vi "Global Log To String.vi"(10 "Log":T1) -> (3 "Log String":string)   [LabVIEW 2017, in "Communicable State Machine.lvlib"]
doc: "Converts global log data clusters to strings.\n\n-- <b>Controls</b> --\n- <b>Log</b>: Global log data cluster.\n\n-- <b>Indicators</b> --\n- <b>Log String</b>: Global log string."
uses:
  Communicable State Machine.lvlib
  _Support/Typedef/_CSM_GlobalLog_MSG.ctl
  _Support/Typedef/_CSM_Response Source Message.ctl
  _Support/Typedef/_CSM_GlobalLog_MSG_TYPE.ctl
  _Shared/CSM Shared.lvlib
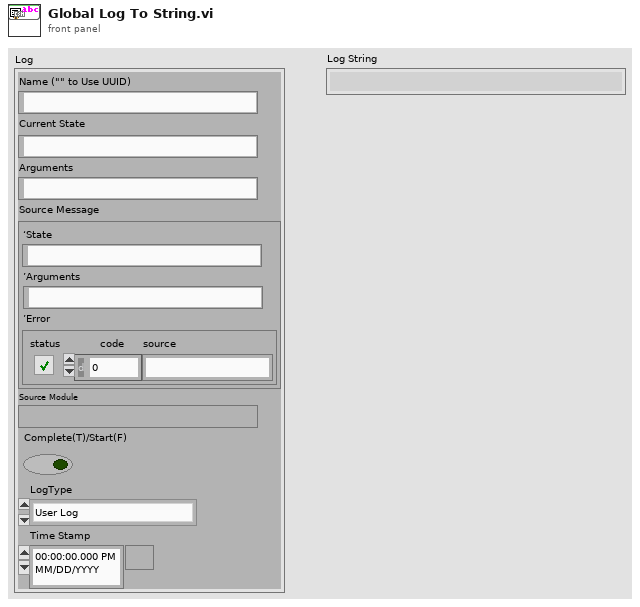
[diagram p1: front panel]
types:
  T1 = typedef "Communicable State Machine.lvlib/_CSM_GlobalLog_MSG.ctl" = cluster{"Name (\"\" to Use UUID)":string, "Current State":string, "Arguments":string, "Source Message":T2, "Source Module":string, "Complete(T)/Start(F)":bool, "LogType":T3, "Time Stamp":timestamp}
  T2 = typedef "Communicable State Machine.lvlib/_CSM_Response Source Message.ctl" = cluster{"‘State":string, "’Arguments":string, "’Error":errorcluster}
  T3 = typedef "Communicable State Machine.lvlib/_CSM_GlobalLog_MSG_TYPE.ctl" = enum16{"User Log", "State Change", "Status", "Interrupt", "Register", "Unregister", "Error Log", "Module Created", "Module Destroyed", "Async Message", "No-Rep Async Message", "Sync Message", "AsyncMsg Complete", "SyncMsg Complete"}
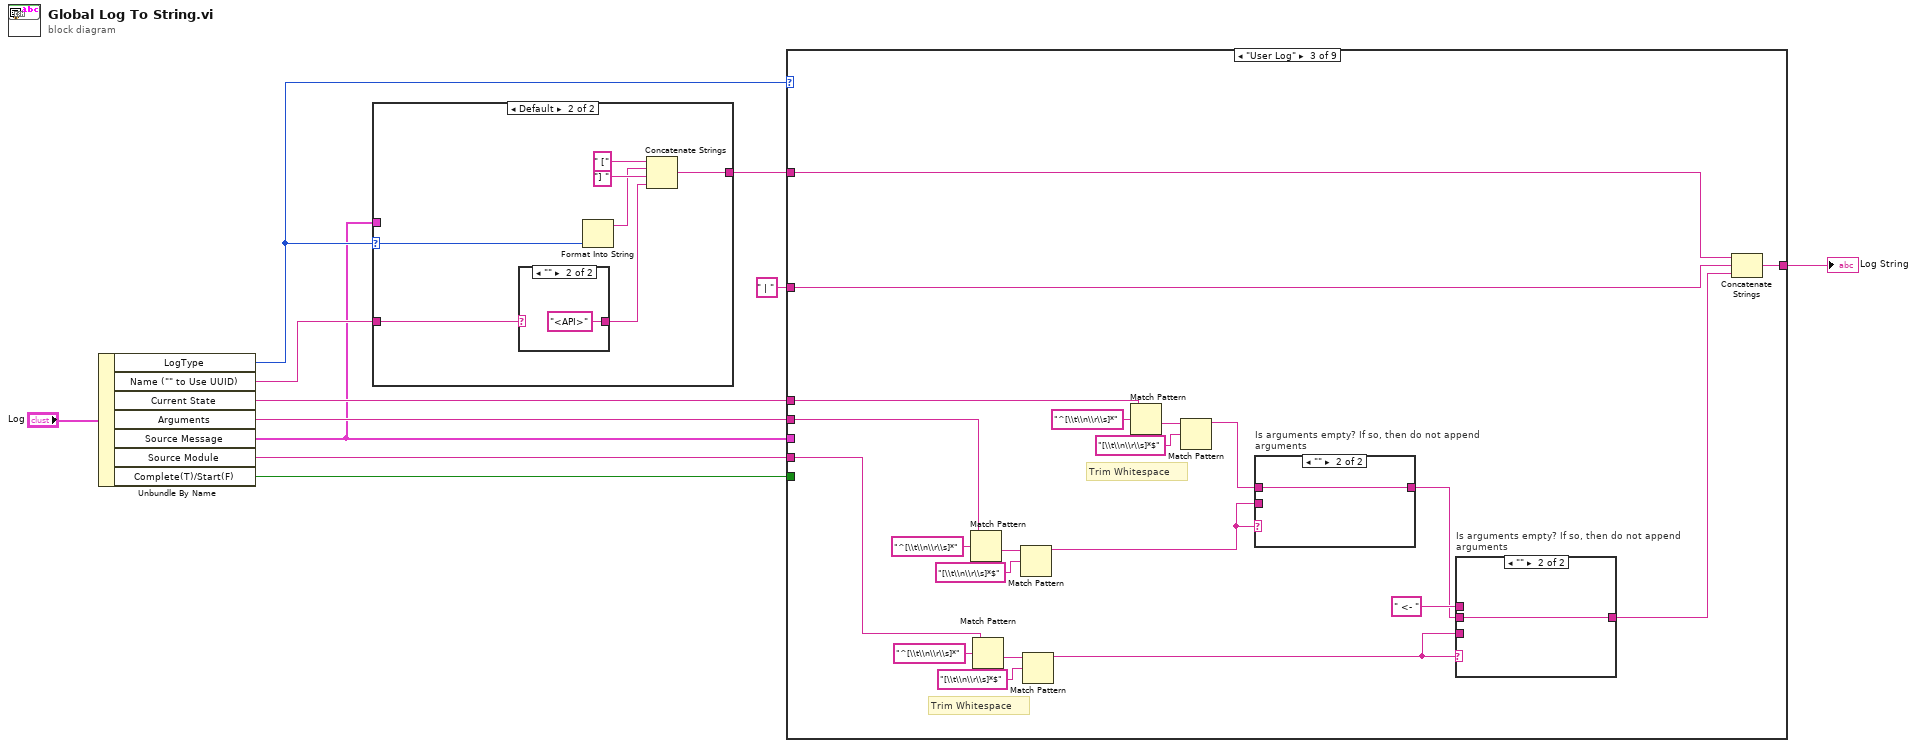
[diagram p0: block diagram]
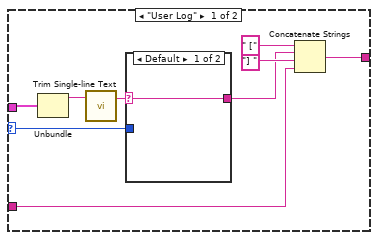
[diagram p2: hidden frame]
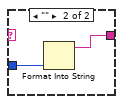
[diagram p3: hidden frame]
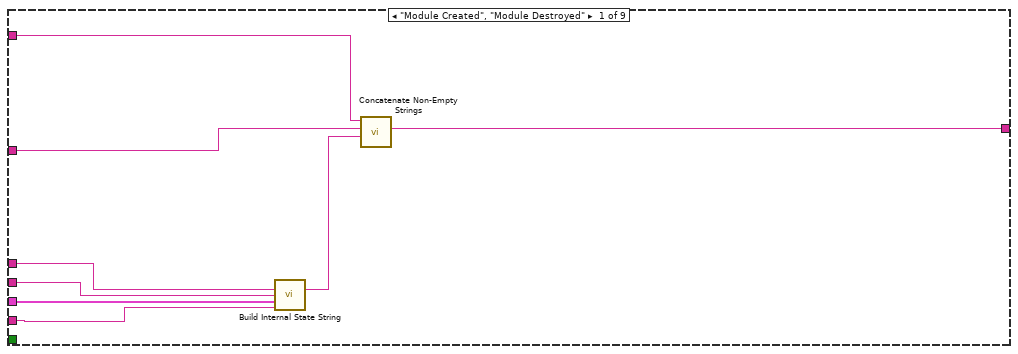
[diagram p5: hidden frame]
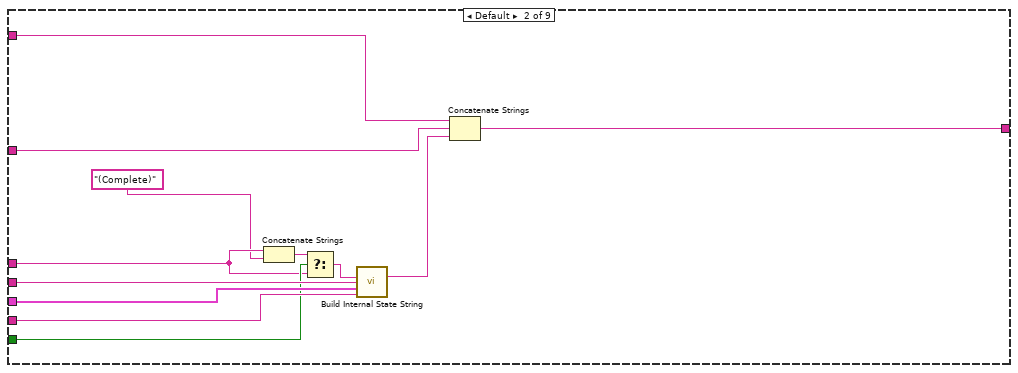
[diagram p6: hidden frame]
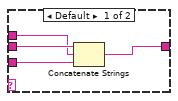
[diagram p7: hidden frame]
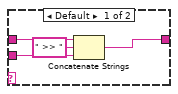
[diagram p8: hidden frame]
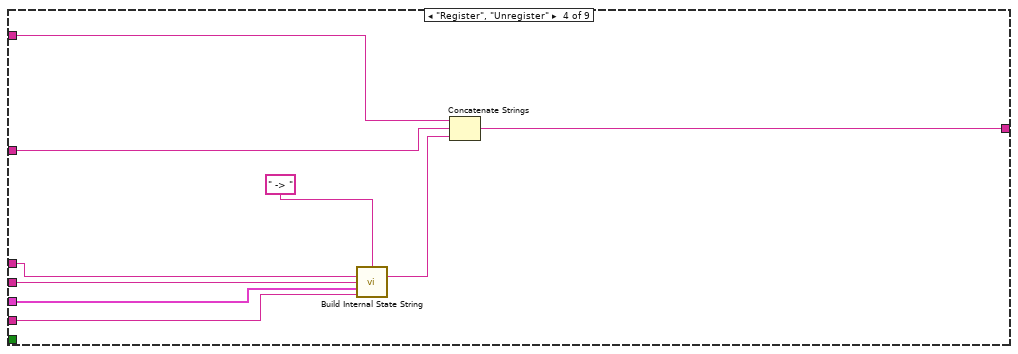
[diagram p9: hidden frame]
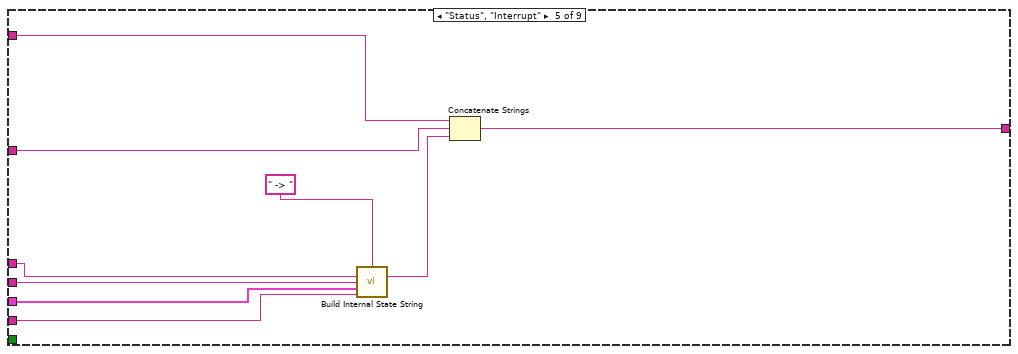
[diagram p10: hidden frame]
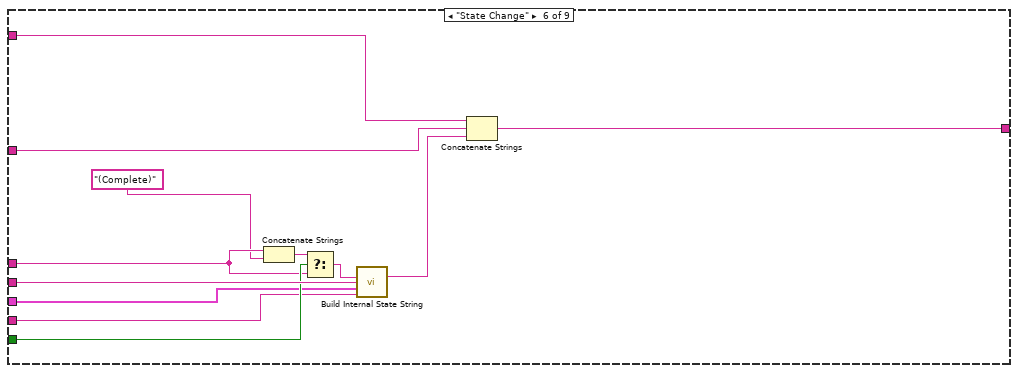
[diagram p11: hidden frame]
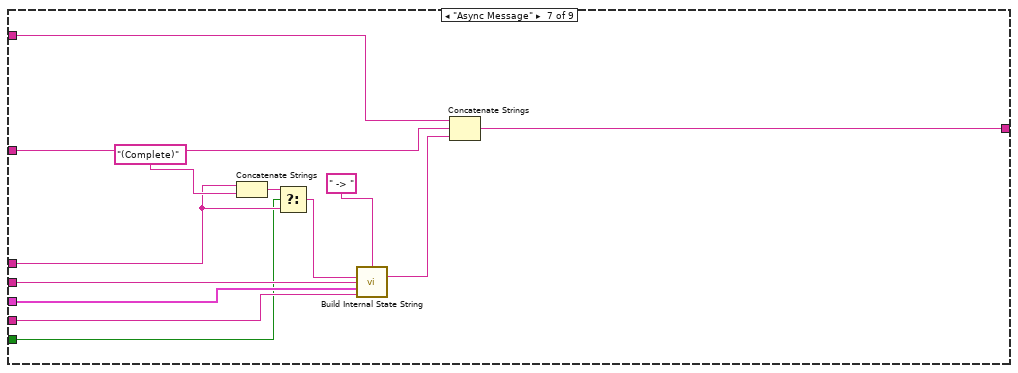
[diagram p12: hidden frame]
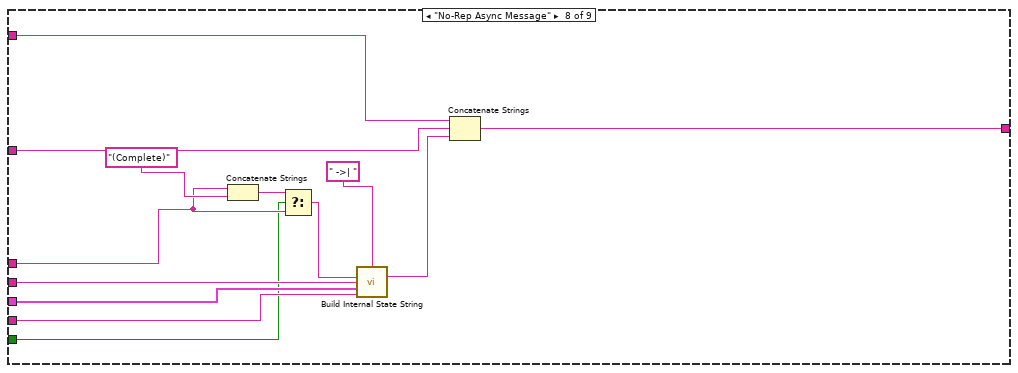
[diagram p13: hidden frame]
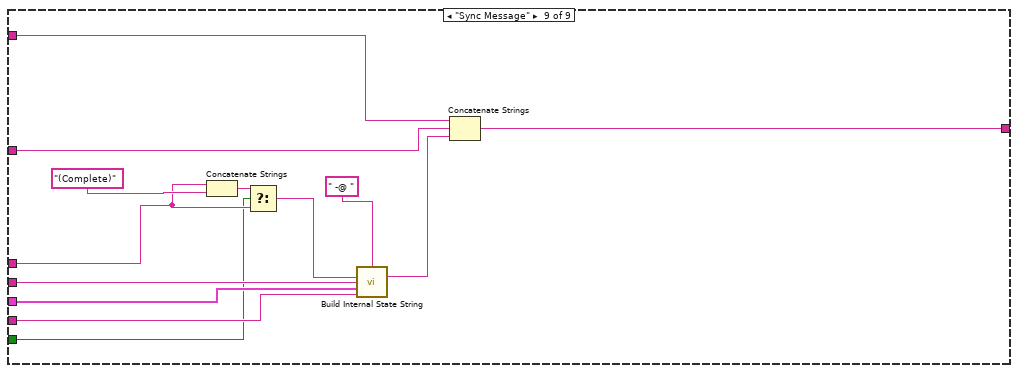
[diagram p14: hidden frame]
diagram:
  n1 = Unbundle By Name("Log") -> ("LogType"=w9:T3, "Name (\"\" to Use UUID)"=w2:string, "Current State"=w5:string, "Arguments"=w7:string, "Source Message"=w1:T2, "Source Module"=w6:string, "Complete(T)/Start(F)"=w4:bool)
  n2 = case shown="Default" w9 {
    selector: w9 -> [w15 w30]
    tunnel: [w17 w26] -> w3
    tunnel: w2 -> [w16 w25]
    tunnel: w1 -> [w13 _]
    frame "User Log" {
      n3 = Unbundle(w13) -> ("‘State"=w14:string)  [unwired: 2 out]
      n4 = call "Trim Single-line Text.vi"("single-line text"=w14) -> ("trimed text"=w12:string)  [unwired: 2 in]
      n5 = case shown="Default" w12 {
        selector: w12 -> [w21 _]
        tunnel: [w21 w23] -> w18
        tunnel: w15 -> [_ w22]
        frame Default {
        }
        frame "" {
          n6 = Format Into String(w22) -> (resulting string=w23:string)  [unwired: 3 in, 1 out]
        }
      }
      n7 = Concatenate Strings(" [" ("string"), w18, "] " ("string"), w16) -> (w17:string)
    }
    frame Default {
      n8 = case shown="\"\"" w25 {
        selector: w25 -> [w31 _]
        tunnel: [w31 "<API>"] -> w24
        frame Default {
        }
        frame "" {
        }
      }
      n9 = Format Into String(w30) -> (resulting string=w27:string)  [unwired: 3 in, 1 out]
      n10 = Concatenate Strings(" [" ("string"), w27, "] " ("string"), w24) -> (w26:string)
    }
  }
  n11 = case shown="\"User Log\"" w9 {
    tunnel: [w39 w52 w73 w92 w101 w113 w126 w139 w152] -> w10
    tunnel: " | " ("string") -> [w40 w51 w72 w91 w100 w112 w125 w138 w151]
    tunnel: w7 -> [w34 w48 w71 w90 w99 w109 w124 w137 w150]
    tunnel: w1 -> [w36 w47 _ w89 w98 w103 w123 w136 w149]
    tunnel: w6 -> [w33 w46 w70 w88 w97 w102 w122 w135 w148]
    tunnel: w5 -> [w35 w44 w69 w87 w96 w107 w116 w129 w142]
    tunnel: w4 -> [_ w45 _ _ _ w108 w114 w127 w140]
    tunnel: w3 -> [w38 w41 w53 w85 w94 w104 w120 w133 w146]
    frame "Module Created", "Module Destroyed" {
      n12 = call "Build Internal State String.vi"("State"=w35, "Arguments (\"\")"=w34, "Additional Information"=w36, "Source (\"\")"=w33) -> ("State With Arguments"=w37:string)  [unwired: 11 in]
      n13 = call "Concatenate Non-Empty Strings.vi"("String2"=w37, "Seperator(Carriage Return)"=w40, "String1"=w38) -> ("Result String"=w39:string)  [unwired: 5 in]
    }
    frame Default {
      n14 = Concatenate Strings(w44, "(Complete)" ("string")) -> (w50:string)
      n15 = Select(t=w50, s=w45, f=w44) -> (s? t:f=w49:string)
      n16 = call "Build Internal State String.vi"("State"=w49, "Arguments (\"\")"=w48, "Additional Information"=w47, "Source (\"\")"=w46) -> ("State With Arguments"=w42:string)  [unwired: 11 in]
      n17 = Concatenate Strings(w41, w51, w42) -> (w52:string)
    }
    frame "User Log" {
      # "Trim Whitespace"
      # "Trim Whitespace"
      n18 = Match Pattern(string=w71, regular expression="^[\\t\\n\\r\\s]*") -> (after substring=w59:string)  [unwired: 1 in, 3 out]
      n19 = Match Pattern(string=w70, regular expression="^[\\t\\n\\r\\s]*") -> (after substring=w63:string)  [unwired: 1 in, 3 out]
      n20 = Match Pattern(string=w59, regular expression="[\\t\\n\\r\\s]*$") -> (before substring=w61:string)  [unwired: 1 in, 3 out]
      n21 = Match Pattern(string=w63, regular expression="[\\t\\n\\r\\s]*$") -> (before substring=w65:string)  [unwired: 1 in, 3 out]
      n22 = Match Pattern(string=w69, regular expression="^[\\t\\n\\r\\s]*") -> (after substring=w55:string)  [unwired: 1 in, 3 out]
      n23 = Match Pattern(string=w55, regular expression="[\\t\\n\\r\\s]*$") -> (before substring=w57:string)  [unwired: 1 in, 3 out]
      n24 = case "Is arguments empty? If so, then do not append arguments" shown="\"\"" w61 {
        tunnel: [w79 w83] -> w66
        tunnel: w57 -> [w82 w83]
        tunnel: w61 -> [w80 _]
        frame Default {
          n25 = Concatenate Strings(w82, " >> " ("string"), w80) -> (w79:string)
        }
        frame "" {
        }
      }
      n26 = case "Is arguments empty? If so, then do not append arguments" shown="\"\"" w65 {
        tunnel: [w75 w78] -> w67
        tunnel: w66 -> [w77 w78]
        tunnel: w65 -> [w76 _]
        tunnel: " <- " ("Seperator(<-)") -> [w74 _]
        frame Default {
          n27 = Concatenate Strings(w77, w74, w76) -> (w75:string)
        }
        frame "" {
        }
      }
      n28 = Concatenate Strings(w53, w72, w67) -> (w73:string)
    }
    frame "Register", "Unregister" {
      n29 = call "Build Internal State String.vi"("Seperator(<-)"=" -> ", "State"=w87, "Arguments (\"\")"=w90, "Additional Information"=w89, "Source (\"\")"=w88) -> ("State With Arguments"=w86:string)  [unwired: 10 in]
      n30 = Concatenate Strings(w85, w91, w86) -> (w92:string)
    }
    frame "Status", "Interrupt" {
      n31 = call "Build Internal State String.vi"("Seperator(<-)"=" -> ", "State"=w96, "Arguments (\"\")"=w99, "Additional Information"=w98, "Source (\"\")"=w97) -> ("State With Arguments"=w95:string)  [unwired: 10 in]
      n32 = Concatenate Strings(w94, w100, w95) -> (w101:string)
    }
    frame "State Change" {
      n33 = Concatenate Strings(w107, "(Complete)" ("string")) -> (w111:string)
      n34 = Select(t=w111, s=w108, f=w107) -> (s? t:f=w110:string)
      n35 = call "Build Internal State String.vi"("State"=w110, "Arguments (\"\")"=w109, "Additional Information"=w103, "Source (\"\")"=w102) -> ("State With Arguments"=w105:string)  [unwired: 11 in]
      n36 = Concatenate Strings(w104, w112, w105) -> (w113:string)
    }
    frame "Async Message" {
      n37 = Concatenate Strings(w116, "(Complete)" ("string")) -> (w118:string)
      n38 = Select(t=w118, s=w114, f=w116) -> (s? t:f=w115:string)
      n39 = call "Build Internal State String.vi"("Seperator(<-)"=" -> ", "State"=w115, "Arguments (\"\")"=w124, "Additional Information"=w123, "Source (\"\")"=w122) -> ("State With Arguments"=w121:string)  [unwired: 10 in]
      n40 = Concatenate Strings(w120, w125, w121) -> (w126:string)
    }
    frame "No-Rep Async Message" {
      n41 = Concatenate Strings(w129, "(Complete)" ("string")) -> (w131:string)
      n42 = Select(t=w131, s=w127, f=w129) -> (s? t:f=w128:string)
      n43 = call "Build Internal State String.vi"("Seperator(<-)"=" ->| ", "State"=w128, "Arguments (\"\")"=w137, "Additional Information"=w136, "Source (\"\")"=w135) -> ("State With Arguments"=w134:string)  [unwired: 10 in]
      n44 = Concatenate Strings(w133, w138, w134) -> (w139:string)
    }
    frame "Sync Message" {
      n45 = Concatenate Strings(w142, "(Complete)" ("string")) -> (w144:string)
      n46 = Select(t=w144, s=w140, f=w142) -> (s? t:f=w141:string)
      n47 = call "Build Internal State String.vi"("Seperator(<-)"=" -@ ", "State"=w141, "Arguments (\"\")"=w150, "Additional Information"=w149, "Source (\"\")"=w148) -> ("State With Arguments"=w147:string)  [unwired: 10 in]
      n48 = Concatenate Strings(w146, w151, w147) -> (w152:string)
    }
  }
  "Log String" <- w10
